vi "Select_Single_ADAM_Ch.vi"(0 "Desired Ch name (in)":string, 3 "Available Ch names":string[](array[string]), 4 "Message":string) -> (6 "Ch Name":string)   [LabVIEW 2010]
panel:
  in  "Choose desired ADAM channels":i32(listbox)
  in  "ok":bool
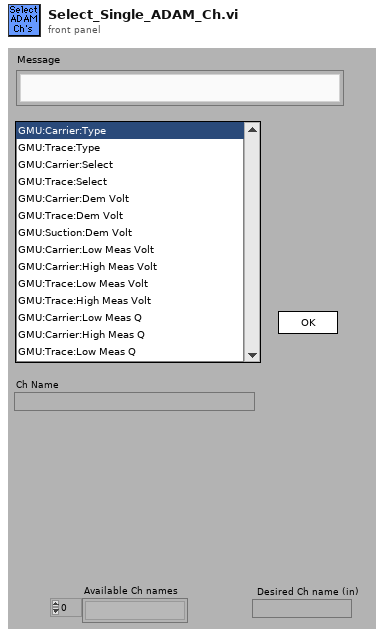
[diagram p1: front panel]
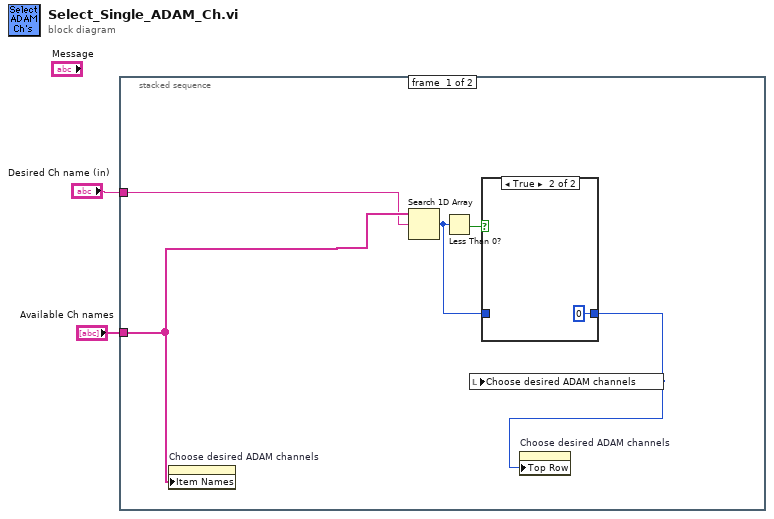
[diagram p0: block diagram]
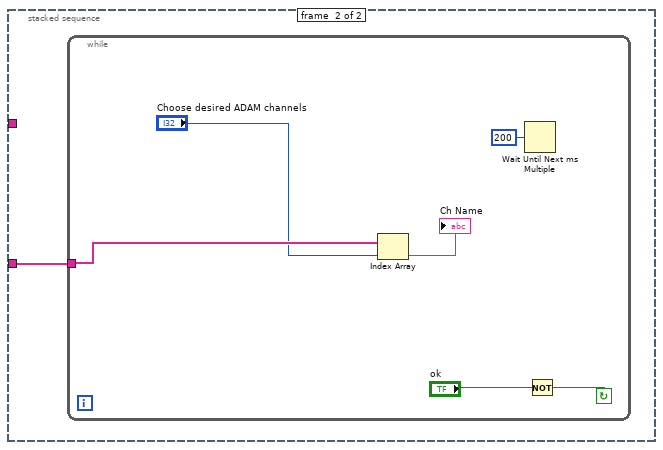
[diagram p3: hidden frame]
diagram:
  n1 = stacked-sequence {
    tunnel: "Available Ch names" -> [w7 w10]
    tunnel: "Desired Ch name (in)" -> [w6 _]
    frame #0 {
      n2 = property on="Choose desired ADAM channels" class="LstBox (strict)"("Item Names"=w7) -> ()  [unwired: 2 in, 2 out]
      n3 = Search 1D Array(1D array=w7, element=w6) -> (index of element=w4:i32)  [unwired: 1 out]
      n4 = Less Than 0?(x=w4) -> (x < 0?=w5:bool)
      n5 = case shown="True" w5 {
        tunnel: w4 -> [w8 _]
        tunnel: [w8 0 ("index of element")] -> w3
        frame False {
        }
        frame True {
        }
      }
      n6 = local write "Choose desired ADAM channels"(w3) -> ()
      n7 = property on="Choose desired ADAM channels" class="LstBox (strict)"("Top Row"=w3) -> ()  [unwired: 2 in, 2 out]
    }
    frame #1 {
      n8 = while {
        tunnel: w10 -> [w13]
        stop <- w15 continue-if-true
        n9 = Index Array(array=w13, index="Choose desired ADAM channels") -> (element=→"Ch Name":string)
        n10 = Wait Until Next ms Multiple(millisecond multiple=u32 200) -> ()  [unwired: 1 out]
        n11 = Not(x="ok") -> (.not. x?=w15:bool)
      }
    }
  }
